vi "read and log co2 levels.vi"() -> ()   [LabVIEW 2013]
panel:
  out "read error":bool
  out "reading":i32
  out "co2 fast":string
  in  "inter-read time (ms)":u32=250
  in  "CO2 meter serial port(s)":refnum<visa-resource-name>[](array[refnum])=["COM4"]
  in  "stop":bool
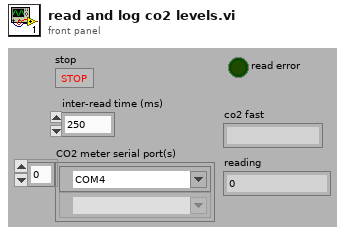
[diagram p1: front panel]
types:
  T1 = enum16{"Reset Table", "Get Values", "Add Value", "Get Table", "Get Spreadsheet"}
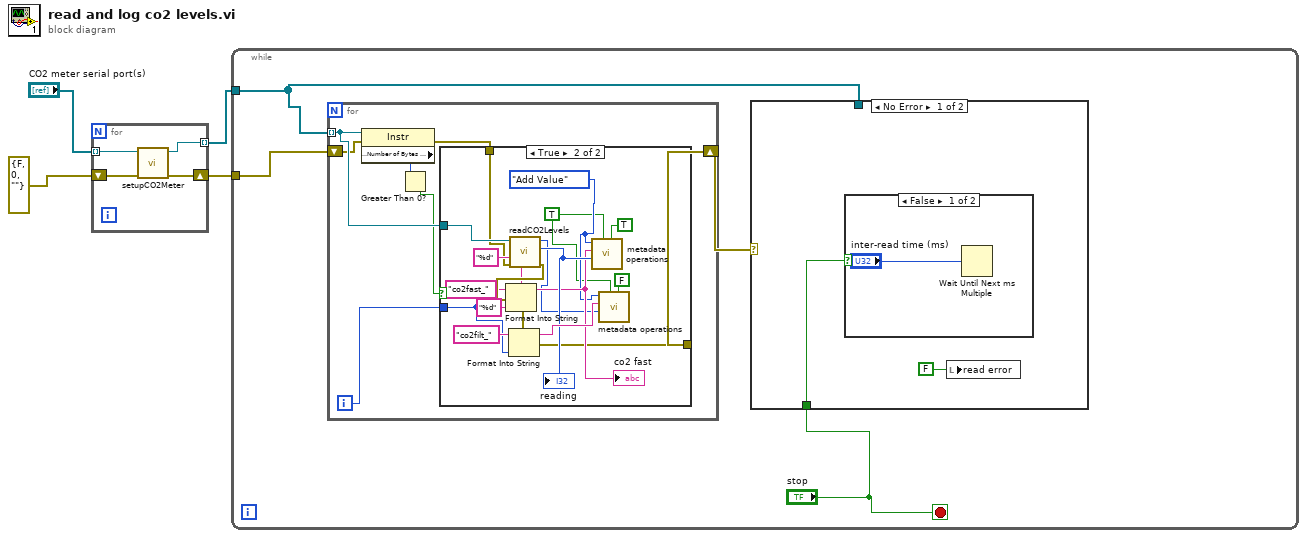
[diagram p0: block diagram]
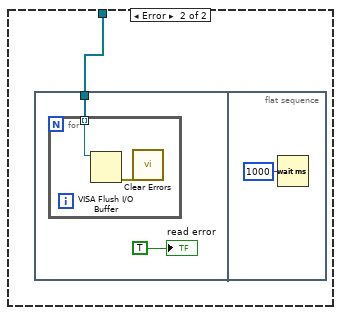
[diagram p3: hidden frame]
diagram:
  n1 = for {
    tunnel: "CO2 meter serial port(s)" -> [w7] mode=indexing
    tunnel: [w6] -> w2 mode=indexing
    shift-right: [w5] -> w1
    shift-left: errorcluster {"status"=FALSE, "code"=0, "source"=""} ("error IO") -> [w8]
    n2 = call "setupCO2Meter.vi"("VISA resource name"=w7, "error in (no error)"=w8) -> ("VISA resource name out"=w6:refnum<visa-resource-name>, "error out"=w5:errorcluster)  [unwired: 7 in]
  }
  n3 = while {
    tunnel: w2 -> [w11]
    tunnel: w1 -> [w10]
    stop <- "stop" stop-if-true
    n4 = for {
      tunnel: w11 -> [w27] mode=indexing
      shift-right: [w24] -> w12
      shift-left: w10 -> [w22]
      i -> [w26]
      n5 = property class="Instr"(reference=w27, error in=w22) -> (error out=w25:errorcluster, "Serial Settings:Number of Bytes at Serial Port"=w28:u32)  [unwired: 1 out]
      n6 = Greater Than 0?(x=w28) -> (x > 0?=w23:bool)
      n7 = case shown="True" w23 {
        tunnel: w27 -> [_ w36]
        tunnel: w26 -> [_ w35]
        tunnel: w25 -> [w29 w34]
        tunnel: [w29 w33] -> w24
        frame False {
        }
        frame True {
          w30 = TRUE ("add to stackreader")
          w32 = T1."Add Value" ("Operation")
          n8 = call "readCO2Levels.vi"("error in (no error)"=w34, "VISA resource name"=w36) -> ("error IO"=w39:errorcluster, "Fast Level"=w44:i32, "Filtered Level"=w31:i32)  [unwired: 7 in]
          "reading" <- w44
          n9 = Format Into String(format string="%d", initial string="co2fast_", error in=w39, w35) -> (resulting string=w43:string, error out=w42:errorcluster)
          "co2 fast" <- w43
          n10 = Format Into String(format string="%d", initial string="co2filt_", error in=w42, w35) -> (resulting string=w45:string, error out=w33:errorcluster)
          n11 = call "metadata operations.vi"("add time?"=TRUE, "add to stack writer"=w30, "value"=w44, "key"=w43, "Operation"=w32) -> ()  [unwired: 3 in, 4 out]
          n12 = call "metadata operations.vi"("add time?"=FALSE, "add to stack writer"=w30, "value"=w31, "key"=w45, "Operation"=w32) -> ()  [unwired: 3 in, 4 out]
        }
      }
    }
    n13 = case shown="No Error" w12 {
      tunnel: w11 -> [_ w16]
      tunnel: "stop" -> [w14 _]
      frame No Error {
        n14 = case shown="False" w14 {
          frame False {
            n15 = Wait Until Next ms Multiple(millisecond multiple="inter-read time (ms)") -> ()  [unwired: 1 out]
          }
          frame True {
          }
        }
        n16 = local write "read error"(FALSE ("read error")) -> ()
      }
      frame Error {
        n17 = flat-sequence {
          tunnel: w16 -> [w18]
          frame #0 {
            n18 = for {
              tunnel: w18 -> [w20] mode=indexing
              n19 = VISA Flush I/O Buffer(VISA resource name=w20) -> (error out=w19:errorcluster)  [unwired: 2 in, 1 out]
              n20 = call <vilib>:"Clear Errors.vi"("error in (no error)"=w19) -> ()  [unwired: 6 in, 1 out]
            }
            "read error" <- TRUE ("read error")
          }
          frame #1 {
            n21 = Wait (ms)(milliseconds to wait=u32 1000) -> ()  [unwired: 1 out]
          }
        }
      }
    }
  }
